vi "procs.setByProcIndexString.vi"(6 "menu in (get)":enum16{"get", "set"}(ring), 7 "procIndex":i32, 8 "error in":errorcluster, 9 "String in":string, 10 "procAttribute":string, 11 "procs in":cluster{"Procedure":variant[]}[](array[cluster])) -> (0 "error out":errorcluster, 1 "String out":string, 3 "procs out":cluster{"Procedure":variant[]}[](array[cluster]))   [LabVIEW 2024]
uses:
  Polymorphics/variantCtrlString.vi
  proc.util.validateParamExist.vi
  <vilib>/Utility/error.llb/Clear Errors.vi
  util.error.create.vi
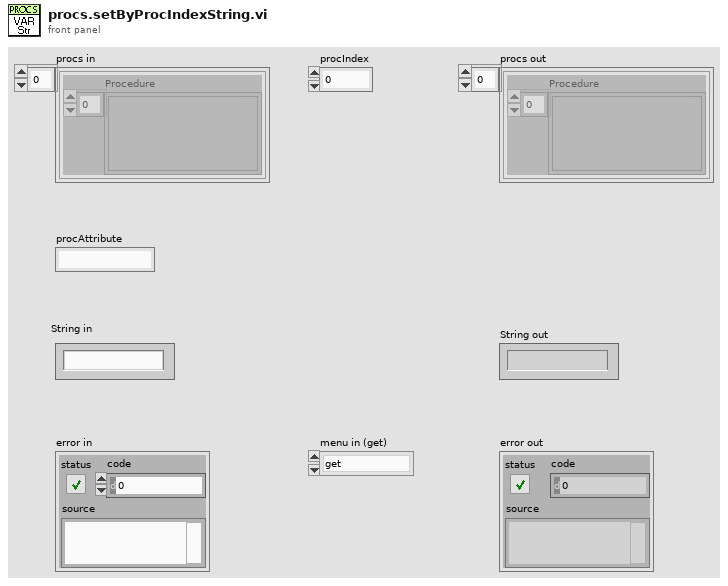
[diagram p1: front panel]
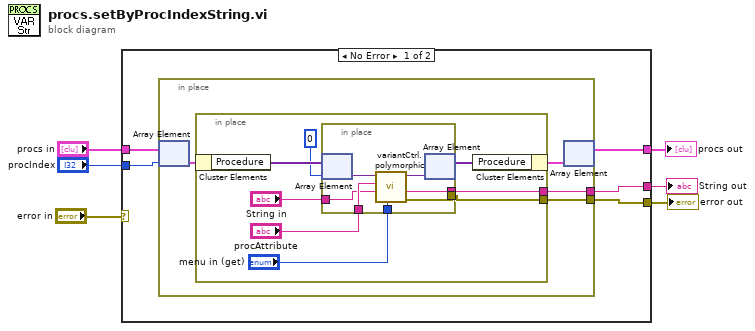
[diagram p0: block diagram]
diagram:
  n1 = case shown="No Error" "error in" {
    selector: "error in" -> [_ w32]
    tunnel: "procIndex" -> [w11 _]
    tunnel: [w10 w31] -> w3
    tunnel: "procs in" -> [w9 w31]
    tunnel: [w8 _] -> w5
    tunnel: [w7 w32] -> w1
    frame No Error {
      n2 = in-place {
        in-place-border: [w13] -> w8
        in-place-border: [w12] -> w7
        n3 = in-place-array #1(w9, w11) -> (w15:cluster{"Procedure":variant[]})
        n4 = in-place {
          in-place-border: [w20] -> w13
          in-place-border: [w19] -> w12
          n5 = in-place-cluster #2(w15) -> ("Procedure"=w23:variant[])
          n6 = in-place {
            in-place-border: [w28] -> w20
            in-place-border: [w27] -> w19
            in-place-border: "procAttribute" -> [w26]
            in-place-border: "menu in (get)" -> [w25]
            in-place-border: "String in" -> [w24]
            n7 = in-place-array #3(w23, 0) -> (w30:variant)
            n8 = call-poly "variantCtrl.polymorphic.vi"("menu in (get)"=w25, "String Value"=w24, "name in"=w26, "Step in"=w30) -> ("error out"=w27:errorcluster, "String Value"=w28:string, "Step out"=w29:variant)  [unwired: 4 in, 1 out]
            n9 = in-place-array #3(w29) -> (w22:variant[])  [unwired: 1 out]
          }
          n10 = in-place-cluster #2("Procedure"=w22) -> (w14:cluster{"Procedure":variant[]})
        }
        n11 = in-place-array #1(w14) -> (w10:cluster{"Procedure":variant[]}[])  [unwired: 1 out]
      }
    }
    frame Error {
    }
  }
  "String out" <- w5
  "procs out" <- w3
  "error out" <- w1
